vi "set PZT minimum.vi"(8 "error in":errorcluster, 11 "Coarse Approach in":refnum<class "Coarse Approach.lvclass">) -> (0 "error out":errorcluster, 3 "Coarse Approach out":refnum<class "Coarse Approach.lvclass">)   [LabVIEW 2020, in "Coarse Approach.lvclass"]
uses:
  Coarse Approach.lvclass
  Coarse Approach.lvclass/Coarse Approach.ctl
  PZT/PZT.lvclass
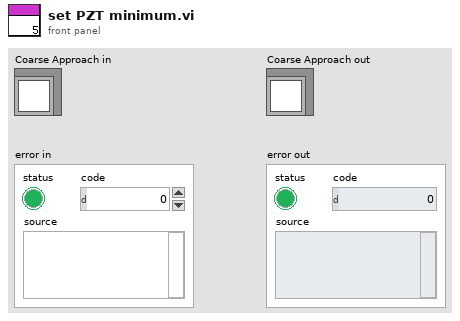
[diagram p1: front panel]
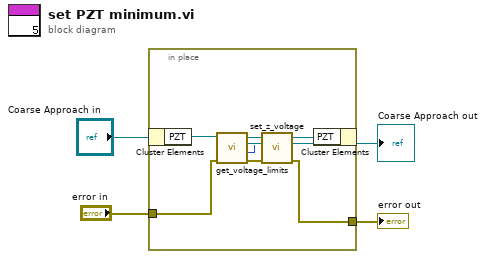
[diagram p0: block diagram]
diagram:
  n1 = in-place {
    in-place-border: "error in" -> [w10]
    in-place-border: [w6] -> w1
    n2 = in-place-cluster #1("Coarse Approach in") -> ("PZT"=w11:refnum<class "PZT.lvclass">)
    n3 = call-dynamic "get_voltage_limits.vi"("error in (no error)"=w10, "PZT in"=w11) -> ("error out"=w7:errorcluster, "minimum voltage (bits)"=w8:i16, "PZT out"=w9:refnum<class "PZT.lvclass">)  [unwired: 6 in, 1 out]
    n4 = call-dynamic "set_z_voltage.vi"("error in (no error)"=w7, "Z voltage (bits)"=w8, "PZT in"=w9) -> ("error out"=w6:errorcluster, "PZT out"=w5:refnum<class "PZT.lvclass">)  [unwired: 7 in]
    n5 = in-place-cluster #1("PZT"=w5) -> (→"Coarse Approach out":refnum<class "Coarse Approach.lvclass">)
  }
  "error out" <- w1
